vi "fpgaMain.vi"() -> ()   [LabVIEW 2012]
panel:
  in  "waitUntilIRQClearedIsTrue":bool=TRUE
  in  "loopPeriod_ticks":u32=40000
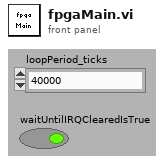
[diagram p1: front panel]
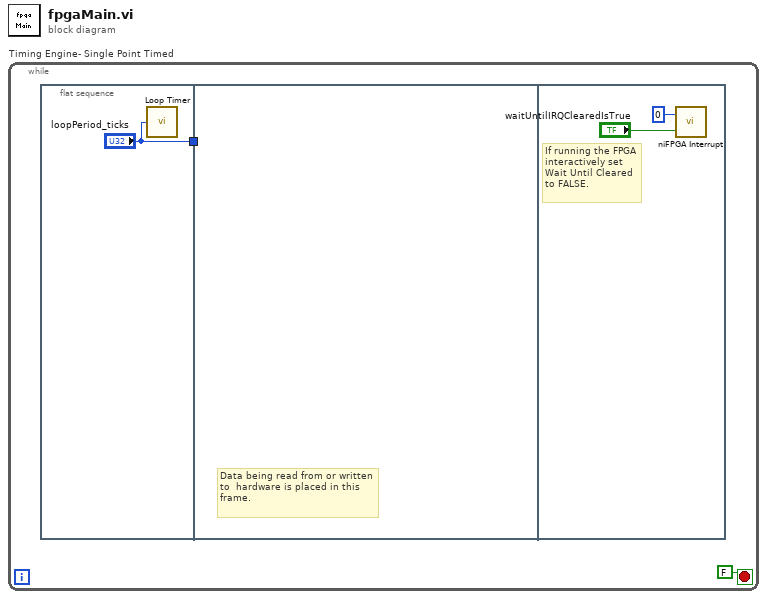
[diagram p0: block diagram]
diagram:
  n1 = while "Timing Engine- Single Point Timed" {
    stop <- FALSE stop-if-true
    n2 = flat-sequence "Data Acquisition Sequence" {
      tunnel: ["loopPeriod_ticks"] -> w1
      tunnel: w1 -> [_]
      frame #0 {
        n3 = call "Loop Timer"("Count(Ticks)"="loopPeriod_ticks") -> ()  [unwired: 1 out]
      }
      frame #1 {
        # "Data being read from or written to  hardware is placed in this frame."
      }
      frame #2 {
        # "If running the FPGA interactively set Wait Until Cleared to FALSE."
        n4 = call <vilib>:"niFPGA Interrupt.vi"("Wait Until Cleared (F)"="waitUntilIRQClearedIsTrue", "IRQ Number (0)"=u8 0 ("IRQBit")) -> ()  [unwired: 1 in]
      }
    }
  }
